vi "Traffic Light Automatic - ENUM, Case Structure & While Loop-Shift Register.vi"() -> ()   [LabVIEW 2016]
panel:
  in  "EMERGENCY STOP":bool
  out "Green":bool
  out "Yellow":bool
  out "Red":bool
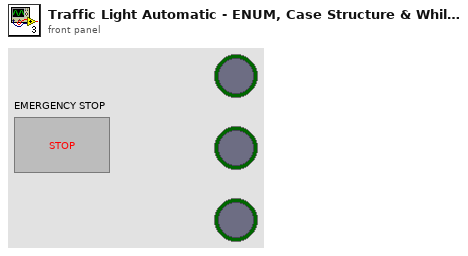
[diagram p1: front panel]
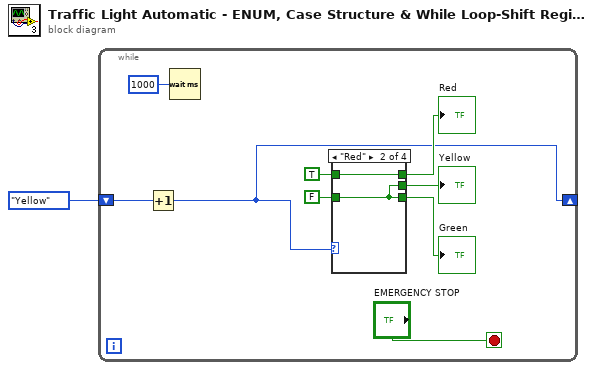
[diagram p0: block diagram]
diagram:
  n1 = while {
    shift-right: [w2] -> _
    shift-left: enum16{"Red", "Yellow", "Green"}."Yellow" ("Enum") -> [w3]
    stop <- "EMERGENCY STOP" stop-if-true
    n2 = Increment(x=w3) -> (x+1=w2:enum16{"Red", "Yellow", "Green"})
    n3 = Wait (ms)(milliseconds to wait=u32 1000) -> ()  [unwired: 1 out]
    n4 = case shown="\"Red\"" w2 {
      tunnel: [w11 w12 w15 w17] -> w10
      tunnel: FALSE -> [w11 w12 w15 w16]
      tunnel: [w11 w13 w15 w16] -> w8
      tunnel: [w11 w12 w14 w16] -> w7
      tunnel: TRUE -> [_ w13 w14 w17]
      frame Default {
      }
      frame "Red" {
      }
      frame "Yellow" {
      }
      frame "Green" {
      }
    }
    "Red" <- w8
    "Yellow" <- w7
    "Green" <- w10
  }
